vi "Disconnect.vi"(8 "error in (no error)":errorcluster, 11 "IVI Oscilloscope in":refnum<class "IVI Oscilloscope.lvclass">) -> (0 "error out":errorcluster, 3 "IVI Oscilloscope out":refnum<class "IVI Oscilloscope.lvclass">)   [LabVIEW 2014, in "IVI Oscilloscope.lvclass"]
uses:
  IVI Oscilloscope.lvclass
  IVI Oscilloscope.lvclass/IVI Oscilloscope.ctl
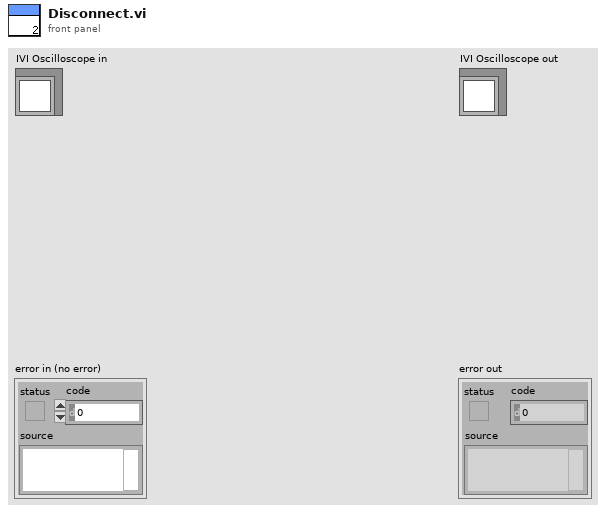
[diagram p1: front panel]
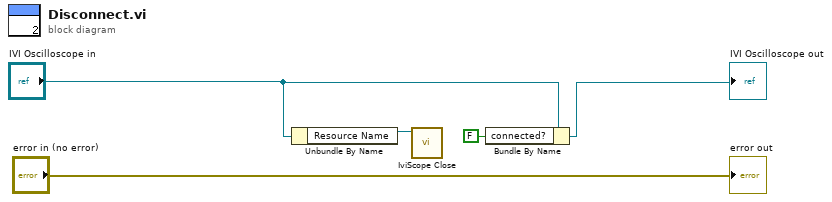
[diagram p0: block diagram]
diagram:
  n1 = Unbundle By Name("IVI Oscilloscope in") -> ("Resource Name"=w5:refnum<k15>)
  n2 = call <vilib>:"IviScope Close.vi"("instrument handle"=w5) -> ()  [unwired: 10 in, 1 out]
  n3 = Bundle By Name(cluster="IVI Oscilloscope in", "connected?"=FALSE) -> (→"IVI Oscilloscope out":refnum<class "IVI Oscilloscope.lvclass">)
  "error out" <- "error in (no error)"
